vi "UsrProfiles-Obtain profile filepath.vi"(8 "error in":errorcluster, 11 "Profile name":string) -> (0 "error out":errorcluster, 3 "Profile filepath":path)   [LabVIEW 2020]
uses:
  Typedefs/Which path.ctl
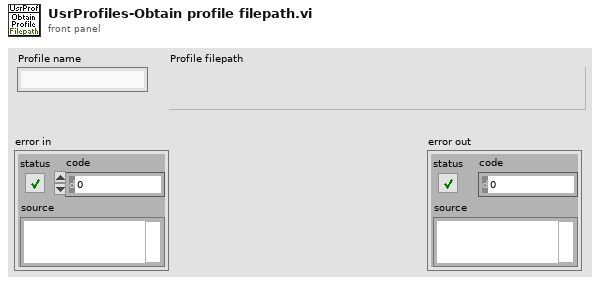
[diagram p1: front panel]
types:
  T1 = typedef "Which path.ctl" = enum16{"Configuration Files", "Calibration Files", "Images", "Setup.ini", "Loaded User profile.ini", "User's-Previous session.ini", "New user profile.ini", "Selected User profile.ini", "User profiles folder", "Power meter scaling.txt", "FOV Cal.ini", "Calibration.ini"}
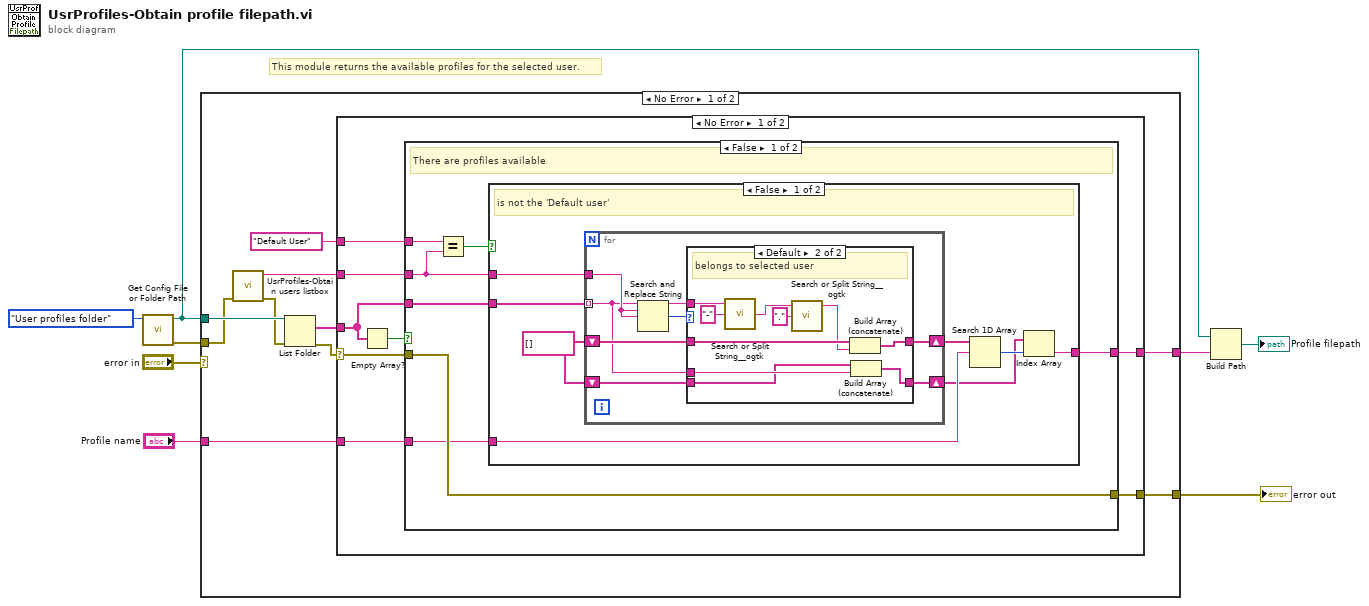
[diagram p0: block diagram]
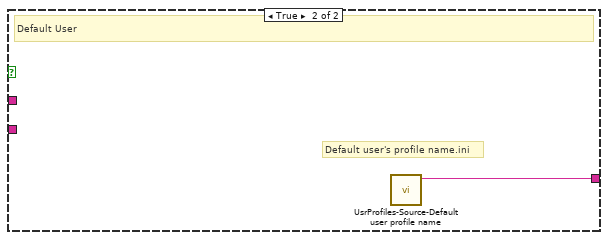
[diagram p3: hidden frame]
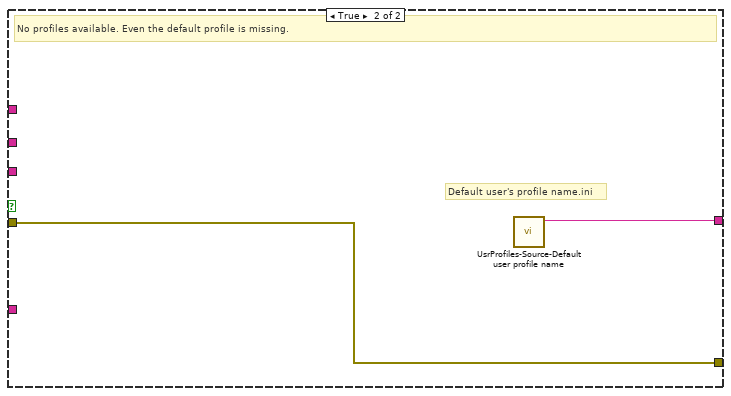
[diagram p4: hidden frame]
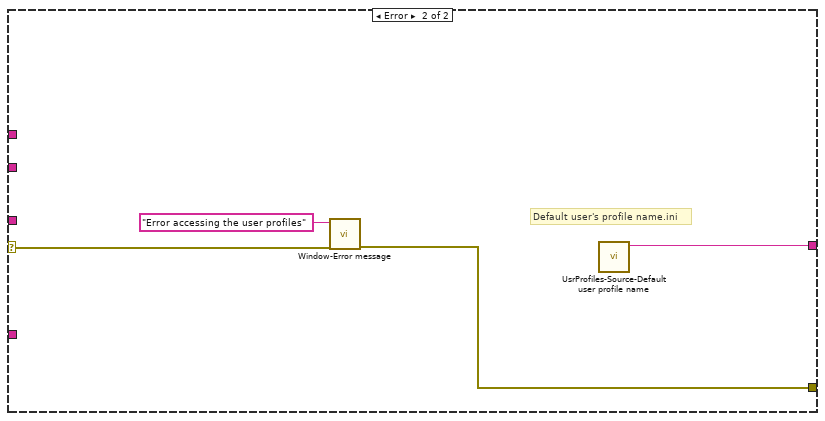
[diagram p5: hidden frame]
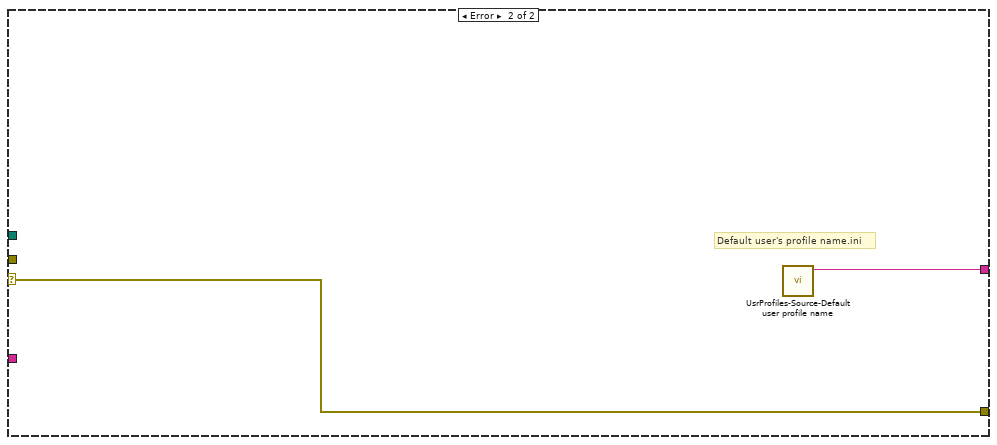
[diagram p6: hidden frame]
diagram:
  # "This module returns the available profiles for the selected user."
  n1 = call "Get Config File or Folder Path.vi"("Which file or folder?"=Which_path."User profiles folder") -> ("Error Out"=w4:errorcluster, "File Path"=w3:path)  [unwired: 8 in, 1 out]
  n2 = case shown="No Error" "error in" {
    selector: "error in" -> [_ w70]
    tunnel: [w16 w70] -> w8
    tunnel: "Profile name" -> [w14 _]
    tunnel: [w13 w69] -> w2
    tunnel: w4 -> [w10 _]
    tunnel: w3 -> [w12 _]
    frame No Error {
      n3 = call "UsrProfiles-Obtain users listbox.vi"("error in (no error)"=w10) -> ("error out"=w9:errorcluster, "Selected user's name"=w11:string)  [unwired: 7 in, 2 out]
      n4 = List Folder(path=w12, error in=w9) -> (filenames=w17:string[], error out=w18:errorcluster)  [unwired: 2 in, 2 out]
      n5 = case shown="No Error" w18 {
        selector: w18 -> [w25 w68]
        tunnel: w17 -> [w23 _]
        tunnel: [w24 w66] -> w16
        tunnel: w11 -> [w22 _]
        tunnel: "Default User" -> [w21 _]
        tunnel: w14 -> [w20 _]
        tunnel: [w19 w65] -> w13
        frame No Error {
          n6 = Empty Array?(array=w23) -> (empty?=w26:bool)
          n7 = case shown="False" w26 {
            tunnel: w23 -> [w33 _]
            tunnel: w25 -> [w32 w64]
            tunnel: [w32 w64] -> w24
            tunnel: w22 -> [w31 _]
            tunnel: w21 -> [w30 _]
            tunnel: w20 -> [w28 _]
            tunnel: [w27 w63] -> w19
            frame False {
              # "There are profiles available"
              n8 = Equal?(x=w30, y=w31) -> (x = y?=w29:bool)
              n9 = case shown="False" w29 {
                tunnel: w33 -> [w41 _]
                tunnel: w31 -> [w40 _]
                tunnel: w28 -> [w37 _]
                tunnel: [w34 w62] -> w27
                frame False {
                  w39 = string[] []
                  # "is not the 'Default user'"
                  n10 = for {
                    tunnel: w41 -> [w44] mode=indexing
                    shift-right: [w48] -> w38
                    shift-left: w39 -> [w49]
                    tunnel: w40 -> [w45]
                    shift-right: [w42] -> w35
                    shift-left: w39 -> [w43]
                    n11 = Search and Replace String(input string=w44, search string=w45, replace string=w45) -> (result string=w47:string, number of replacements=w46:i32)  [unwired: 5 in, 2 out]
                    n12 = case shown="Default" w46 {
                      tunnel: w49 -> [w51 w60]
                      tunnel: [w51 w59] -> w48
                      tunnel: w47 -> [_ w58]
                      tunnel: w44 -> [_ w54]
                      tunnel: w43 -> [w50 w53]
                      tunnel: [w50 w52] -> w42
                      frame 0 {
                      }
                      frame Default {
                        # "belongs to selected user"
                        n13 = call <userlib>:"Search or Split String__ogtk.vi"("search string/char (-)"="-", "string"=w58) -> ("substring after match"=w56:string)  [unwired: 1 in, 2 out]
                        n14 = call <userlib>:"Search or Split String__ogtk.vi"("search string/char (-)"=".", "string"=w56) -> ("substring before match"=w55:string)  [unwired: 1 in, 2 out]
                        n15 = Build Array (concatenate)(w60, w55) -> (w59:string[])
                        n16 = Build Array (concatenate)(w53, w54) -> (w52:string[])
                      }
                    }
                  }
                  n17 = Search 1D Array(1D array=w38, element=w37) -> (index of element=w36:i32)  [unwired: 1 in]
                  n18 = Index Array(array=w35, index=w36) -> (element=w34:string)
                }
                frame True {
                  # "Default user's profile name.ini"
                  # "Default User"
                  n19 = call "UsrProfiles-Source-Default user profile name.vi"() -> ("Default user's profile file name & extension"=w62:string)  [unwired: 11 in]
                }
              }
            }
            frame True {
              # "Default user's profile name.ini"
              # "No profiles available. Even the default profile is missing."
              n20 = call "UsrProfiles-Source-Default user profile name.vi"() -> ("Default user's profile file name & extension"=w63:string)  [unwired: 11 in]
            }
          }
        }
        frame Error {
          # "Default user's profile name.ini"
          n21 = call "Window-Error message.vi"("error in (no error)"=w68, "Message"="Error accessing the user profiles") -> ("Error Out (no error)"=w66:errorcluster)  [unwired: 9 in]
          n22 = call "UsrProfiles-Source-Default user profile name.vi"() -> ("Default user's profile file name & extension"=w65:string)  [unwired: 11 in]
        }
      }
    }
    frame Error {
      # "Default user's profile name.ini"
      n23 = call "UsrProfiles-Source-Default user profile name.vi"() -> ("Default user's profile file name & extension"=w69:string)  [unwired: 11 in]
    }
  }
  "error out" <- w8
  n24 = Build Path(base path=w3, name or relative path=w2) -> (appended path=→"Profile filepath":path)
